vi "Check State-Value Table.vi"(8 "error in (no error)":errorcluster, 9 "State Values":i32[](array[numeric]), 10 "State Names":string[](array[string]), 11 "Channel Ref in":T1 format="%.0x") -> (0 "error out":errorcluster, 3 "Channel Ref out":T1=18446744073709551615 format="%.0x")   [LabVIEW 2017, in "Routing and Faulting Scripting.lvlib"]
uses:
  Routing and Faulting Scripting.lvlib
  <vilib>/NI Veristand/Custom Device API/Custom Device Item Ref.ctl
  <vilib>/NI VeriStand/Custom Device API/Custom Device API.lvlib
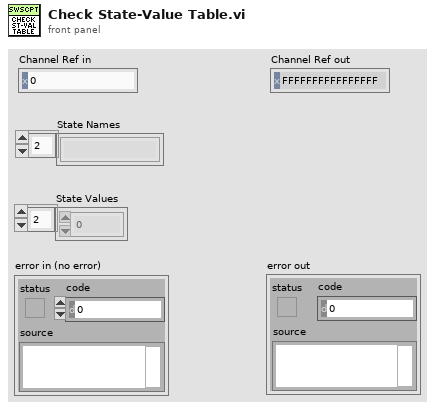
[diagram p1: front panel]
types:
  T1 = typedef "Custom Device API.lvlib/Custom Device Item Ref.ctl" = u64
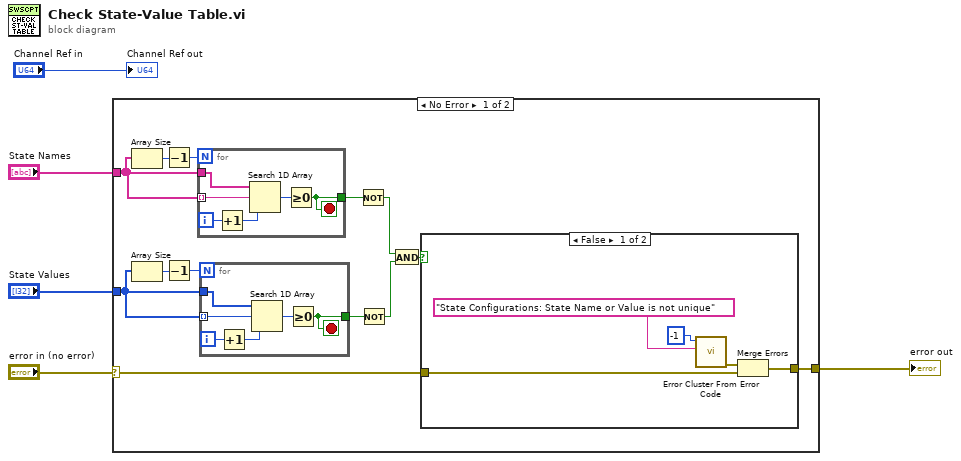
[diagram p0: block diagram]
diagram:
  n1 = case shown="No Error" "error in (no error)" {
    selector: "error in (no error)" -> [w18 w37]
    tunnel: [w17 w37] -> w4
    tunnel: "State Names" -> [w12 _]
    tunnel: "State Values" -> [w6 _]
    frame No Error {
      n2 = Array Size(array=w12) -> (size(s)=w10:i32)
      n3 = Array Size(array=w6) -> (size(s)=w8:i32)
      n4 = Decrement(x=w10) -> (x-1=w11:i32)
      n5 = Decrement(x=w8) -> (x-1=w7:i32)
      n6 = for {
        N: w11 -> [_]
        tunnel: [w35] -> w15
        tunnel: w12 -> [w33] mode=indexing
        tunnel: w12 -> [w32]
        i -> [w34]
        stop <- w35 stop-if-true
        n7 = Increment(x=w34) -> (x+1=w31:i32)
        n8 = Search 1D Array(1D array=w32, element=w33, start index (0)=w31) -> (index of element=w36:i32)
        n9 = Greater Or Equal To 0?(x=w36) -> (x >= 0?=w35:bool)
      }
      n10 = for {
        N: w7 -> [_]
        tunnel: [w23] -> w9
        tunnel: w6 -> [w21] mode=indexing
        tunnel: w6 -> [w20]
        i -> [w22]
        stop <- w23 stop-if-true
        n11 = Increment(x=w22) -> (x+1=w19:i32)
        n12 = Search 1D Array(1D array=w20, element=w21, start index (0)=w19) -> (index of element=w24:i32)
        n13 = Greater Or Equal To 0?(x=w24) -> (x >= 0?=w23:bool)
      }
      n14 = Not(x=w15) -> (.not. x?=w14:bool)
      n15 = Not(x=w9) -> (.not. x?=w13:bool)
      n16 = And(x=w14, y=w13) -> (x .and. y?=w16:bool)
      n17 = case shown="False" w16 {
        tunnel: w18 -> [w26 w30]
        tunnel: [w25 w30] -> w17
        frame False {
          n18 = call <vilib>:"Error Cluster From Error Code.vi"("error message (\"\")"="State Configurations: State Name or Value is not unique" ("error message (\"\")"), "error code (0)"=-1) -> ("error out"=w27:errorcluster)  [unwired: 7 in]
          n19 = Merge Errors(w27, w26) -> (w25:errorcluster)
        }
        frame True {
        }
      }
    }
    frame Error {
    }
  }
  "error out" <- w4
  "Channel Ref out" <- "Channel Ref in"
